vi "Update image display using selected plane.vi"(8 "error in (no error)":errorcluster) -> (0 "error out":errorcluster)   [LabVIEW 2013]
uses:
  Globals/gl_ROI Entry UI globals.vi
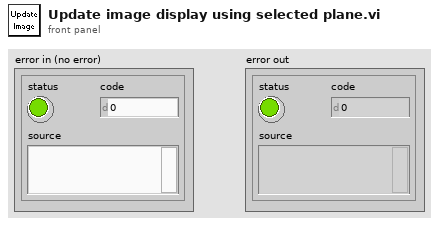
[diagram p1: front panel]
types:
  T1 = typedef "ROI entry screen ctrl refs cluster.ctl" = cluster{"Done button":refnum<vi>, "Imaging button":refnum<vi>, "Acquisition button":refnum<vi>, "POI dwell time (us)":refnum<vi>, "Scan dwell time per pixel (us)":refnum<vi>, "# of planes":refnum<vi>, "Zoom":refnum<vi>, "Equal size":refnum<vi>, "Channel":refnum<vi>, "Image Display":refnum<vi>, "Z-Plane Selector":refnum<vi>, "Number of lines left":refnum<vi>, "Z-stack folder path":refnum<vi>, "POI Density":refnum<vi>, "Arb Plane Entry":refnum<vi>, "Whole plane":refnum<vi>, "Clear Last":refnum<vi>, "Clear All":refnum<vi>, "Trial Length (sec)":refnum<vi>, "Palette Type":refnum<vi>, "Intensity slider":refnum<vi>, "# POI":refnum<vi>, "Max Z Proj":refnum<vi>, "Zplane ind":refnum<vi>, "Wavelength (nm)":refnum<vi>, "Number of Trials":refnum<vi>, "Funct stim.trig.enable":refnum<vi>, "Funct stim.trig.delay (s)":refnum<vi>, "Line Mode":refnum<vi>, "Step size (µm)":refnum<vi>, "ROI move mode":refnum<vi>, "Cool-down time (s)":refnum<vi>, "Enable cool-down time":refnum<vi>, "Motor Z ind. (um)":refnum<vi>, "AOL Z ind. (um)":refnum<vi>}
  T2 = typedef "IMAQ Image.ctl" = refnum<image>
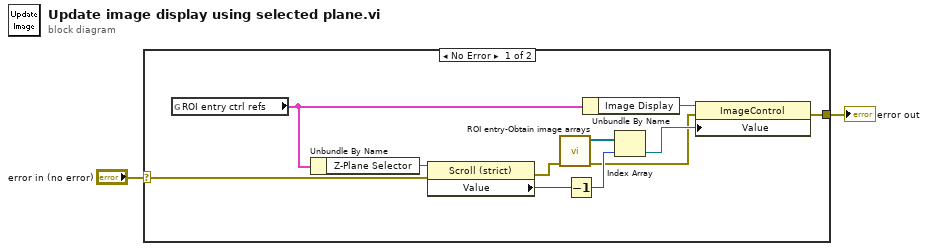
[diagram p0: block diagram]
diagram:
  n1 = case shown="No Error" "error in (no error)" {
    selector: "error in (no error)" -> [w3 w14]
    tunnel: [w6 w14] -> w2
    frame No Error {
      n2 = global read "gl_ROI Entry UI globals.vi" "ROI entry ctrl refs"() -> (w11:T1)
      n3 = Unbundle By Name(w11) -> ("Z-Plane Selector"=w12:refnum<vi>)
      n4 = property on="Property Node" class="Scroll (strict)"(reference=w12, error in=w3) -> (error out=w5:errorcluster, "Value"=w9:i32)  [unwired: 1 out]
      n5 = call "ROI entry-Obtain image arrays.vi"("error in (no error)"=w5) -> ("error IO"=w4:errorcluster, "RedImageArray"=w7:T2[])  [unwired: 9 in]
      n6 = Decrement(x=w9) -> (x-1=w10:i32)
      n7 = Unbundle By Name(w11) -> ("Image Display"=w13:refnum<vi>)
      n8 = Index Array(array=w7, index=w10) -> (element=w8:T2)
      n9 = property on="Property Node" class="ImageControl"(reference=w13, error in=w4, "Value"=w8) -> (error out=w6:errorcluster)  [unwired: 1 out]
    }
    frame Error {
    }
  }
  "error out" <- w2
